vi "Write Serialized Configuration Parameter.vi"(8 "error in (no error)":errorcluster, 10 "Serialized Configuration":string, 11 "ADAS PE Template in":refnum<class "ADAS PE Template.lvclass">) -> (0 "error out":errorcluster, 3 "ADAS PE Template out":refnum<class "ADAS PE Template.lvclass">)   [LabVIEW 2020, in "ADAS PE Template.lvlib" / "ADAS PE Template.lvclass"]
doc: "<b>Write Serialized Configuration Parameter</b>\nThis method writes the serialized configuration data to th class data in the plugin."
uses:
  ADAS PE Template.lvclass
  C:/Program Files/National Instruments/LabVIEW 2020/vi.lib/FlexLogger/SDK/PluginSDK.lvlibp/PEFClasses/SDK/Processing Element/Processing Element.lvclass
  <vilib>/FlexLogger/SDK/PluginSDK.lvlibp/PEFClasses/SDK/Processing Element/Read Parameters Property.vi
  <vilib>/FlexLogger/SDK/PluginSDK.lvlibp/PEFClasses/SDK/Parameters/SetParameter(String).vi
  <vilib>/FlexLogger/SDK/PluginSDK.lvlibp/PEFClasses/SDK/Processing Element/Write Parameters Property.vi
  <vilib>/FlexLogger/SDK/PluginSDK.lvlibp/PEFClasses/SDK/Parameters/Parameters.lvclass
panel:
  # "#via_ignore"
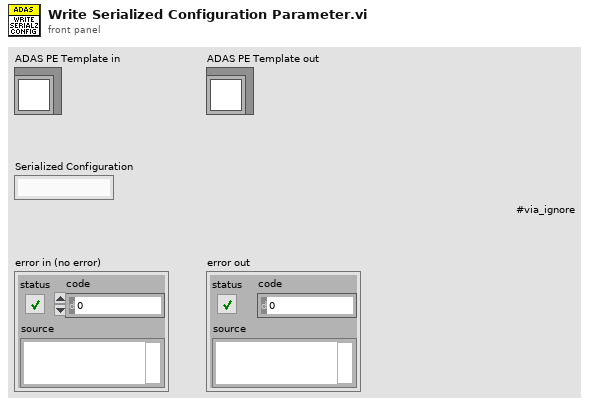
[diagram p1: front panel]
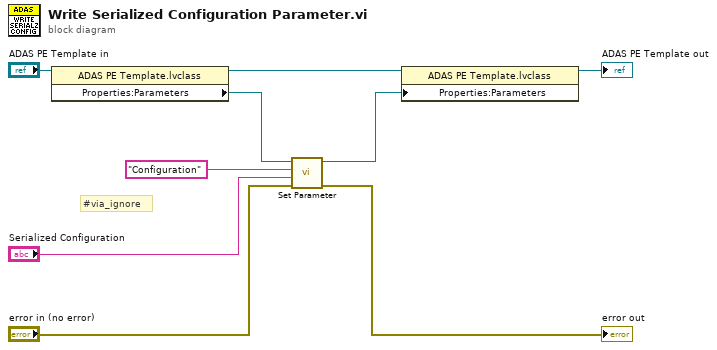
[diagram p0: block diagram]
diagram:
  # "#via_ignore"
  n1 = property on="Property Node" class="ADAS PE Template.lvclass"(reference="ADAS PE Template in") -> (reference out=w5:refnum<class "ADAS PE Template.lvclass">, "Properties:Parameters"=w6:refnum<class "Parameters.lvclass">)  [unwired: 1 in, 1 out]
  n2 = call-poly <vilib>:"Set Parameter.vi"("error in (no error)"="error in (no error)", "Value"="Serialized Configuration", "Name"="Configuration", "Parameters in"=w6) -> ("error out"=→"error out":errorcluster, "Parameters out"=w1:refnum<class "Parameters.lvclass">)  [unwired: 6 in]
  n3 = property on="Property Node" class="ADAS PE Template.lvclass"(reference=w5, "Properties:Parameters"=w1) -> (reference out=→"ADAS PE Template out":refnum<class "ADAS PE Template.lvclass">)  [unwired: 1 in, 1 out]
